vi "Untitled 4.vi"() -> ()   [LabVIEW 2021]
panel:
  in  "y 3":dbl
  in  "y 2":dbl
  in  "y":dbl
  in  "stop":bool
  out "XY Graph":cluster{i32[], dbl[]}[](graph)
  in  "Period":dbl
  in  "SetPoint":dbl
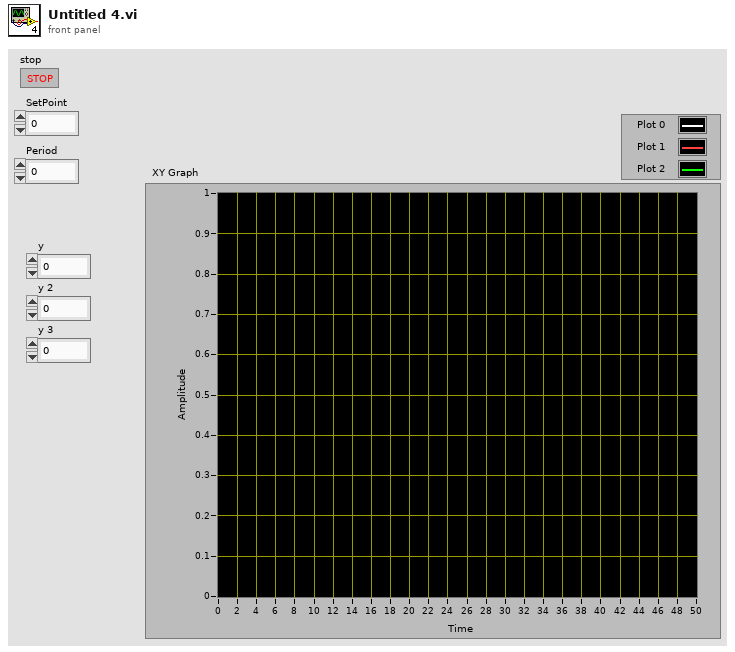
[diagram p1: front panel]
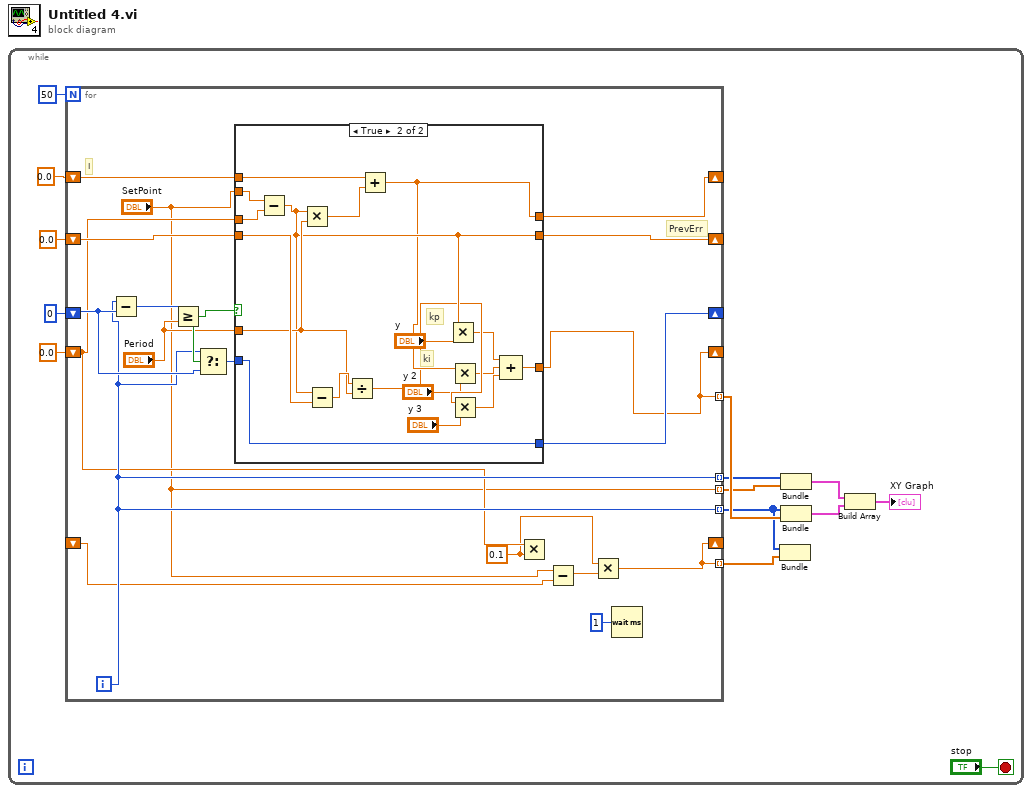
[diagram p0: block diagram]
diagram:
  n1 = while {
    stop <- "stop" stop-if-true
    n2 = for {
      N: 50 -> [_]
      shift-right: [w32] -> _
      shift-left: 0 -> [w26]
      shift-right: [w15] -> _
      shift-left: 0.0 -> [w21]
      shift-right: [w31] -> _
      shift-left: 0.0 -> [w30]
      shift-right: [w28] -> _
      shift-left: 0.0 -> [w29]
      tunnel: [w24] -> w2 mode=indexing
      tunnel: [w15] -> w8 mode=indexing
      tunnel: [w24] -> w7 mode=indexing
      tunnel: ["SetPoint"] -> w6 mode=indexing
      shift-right: [w16] -> _
      shift-left: _ -> [w19]
      tunnel: [w16] -> w1 mode=indexing
      i -> [w24]
      w17 = 0.1 ("y")
      # "PrevErr"
      # "I"
      n3 = Subtract(x=w24, y=w26) -> (x-y=w33:i32)
      n4 = Greater Or Equal?(x=w33, y="Period") -> (x >= y?=w27:bool)
      n5 = Select(t=w24, s=w27, f=w26) -> (s? t:f=w25:i32)
      n6 = case shown="True" w27 {
        tunnel: [w34 w41] -> w32
        tunnel: "SetPoint" -> [_ w55]
        tunnel: w21 -> [w36 w54]
        tunnel: "Period" -> [_ w49]
        tunnel: [w37 w47] -> w31
        tunnel: w30 -> [w37 w53]
        tunnel: w29 -> [w35 w51]
        tunnel: [w35 w48] -> w28
        tunnel: [w36 w42] -> w15
        tunnel: w25 -> [w34 w41]
        frame False {
        }
        frame True {
          # "ki"
          # "kp"
          n7 = Subtract(x=w55, y=w54) -> (x-y=w48:dbl)
          n8 = Multiply(x=w48, y=w49) -> (x*y=w52:dbl)
          n9 = Subtract(x=w48, y=w51) -> (x-y=w50:dbl)
          n10 = Divide(x=w50, y=w49) -> (x/y=w46:dbl)
          n11 = Add(x=w53, y=w52) -> (x+y=w47:dbl)
          n12 = Multiply(x=w48, y="y") -> (x*y=w45:dbl)
          n13 = Multiply(x=w47, y="y 2") -> (x*y=w44:dbl)
          n14 = Multiply(x=w46, y="y 3") -> (x*y=w43:dbl)
          n15 = Compound Arithmetic op=ADD(w45, w44, w43) -> (w42:dbl)
        }
      }
      n16 = Multiply(x=w21, y=w17) -> ()  [unwired: 1 out]
      n17 = Subtract(x="SetPoint", y=w19) -> (x-y=w18:dbl)
      n18 = Multiply(x=w17, y=w18) -> (x*y=w16:dbl)
      n19 = Wait (ms)(milliseconds to wait=u32 1) -> ()  [unwired: 1 out]
    }
    n20 = Bundle(w2, w1) -> ()  [unwired: 1 in, 1 out]
    n21 = Bundle(w7, w6) -> (w5:cluster{i32[], dbl[]})  [unwired: 1 in]
    n22 = Bundle(w2, w8) -> (w9:cluster{i32[], dbl[]})  [unwired: 1 in]
    n23 = Build Array(w5, w9) -> (→"XY Graph":cluster{i32[], dbl[]}[])
  }
